vi "Serial RW.vi"(2 "Porta Serial":refnum<visa-resource-name>="COM7", 3 "Escrita":string, 4 "Função":u8) -> (0 "TemDado":bool, 1 "Leitura":string)   [LabVIEW 2012]
doc: "The Basic Serial Read and Write example performs a Serial Port Read, a Serial Port Write, or a combination of these actions. The user selects the actions (read or write) on the front panel. If both are selected, the VI will write the data first, read data, and then close the VISA session that is opened to the port. This VI will wait until the specified number of bytes is received at the port. Only the number of bytes specified will be read.\n\nINSTRUCTIONS:\n1) Select the serial resource and configuration parameters (baud rate, data bits, parity, stop bits, flow control).\n2) Select the operations to be performed. \n3) Connect the serial port to your device. If no device is available, perform a loopback test by doing one of the following. Short pins 2 and 3 on a RS-232 cable or short pin 4 to pin 8 and pin 5 to pin 9 on a RS-485/422 cable. \n4) Run the VI to see the data read. (The \"read string\" will match the \"string to write\" if a loopback test was performed.)\n\nNote: The parameters set for the serial port must match the parameters of the connected instrument or device. In this example, the bytes to read parameter specifies the number of bytes that the serial port reads. If there were more bytes at the port than the number specified in bytes to read, those bytes would not be read. Also, if you specify to read more bytes than the number of bytes actually read, you might receive a timeout error message.\n\nOn the block diagram, the Configure Serial Port VI sets the configuration parameters. The front panel displays the controls used to configure the basic parameters, such as baud rate, data bits, and parity. Constants configure the other parameters the user probably does not need set. After the VISA Configure Serial Port VI opens the VISA session and configures the port, the VI passes the VISA resource name to other VIs that perform operations on that VISA resource. The VISA Write function sends a command to the serial device and the VISA Read function returns data based on the command. The VISA Close function then closes the reference to the serial device. It is important to close the reference; otherwise communication through with that port through protocols other than VISA might not be possible."
uses:
  <vilib>/Instr/_visa.llb/VISA Configure Serial Port (Instr).vi
panel:
  out "bytes read":u32
  in  "error in":errorcluster
  in  "flow control":u16(ring) items=["None"=0, "XON/XOFF"=1, "RTS/CTS"=2, "DTR/DSR"=4]
  in  "stop bits":u16(ring)=10 items=["1.0"=10, "1.5"=15, "2.0"=20]
  in  "parity":u16(ring) items=["None", "Odd", "Even", "Mark", "Space"]
  in  "data bits":u16=8 min=5 max=8 step=1
  in  "baud rate":u32=9600
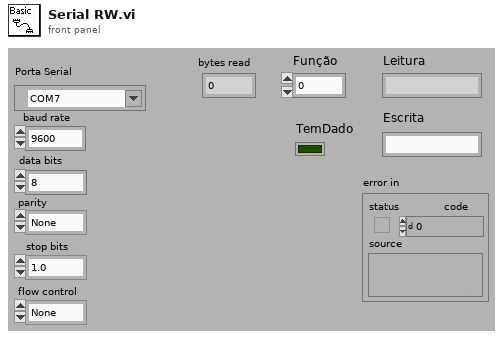
[diagram p1: front panel]
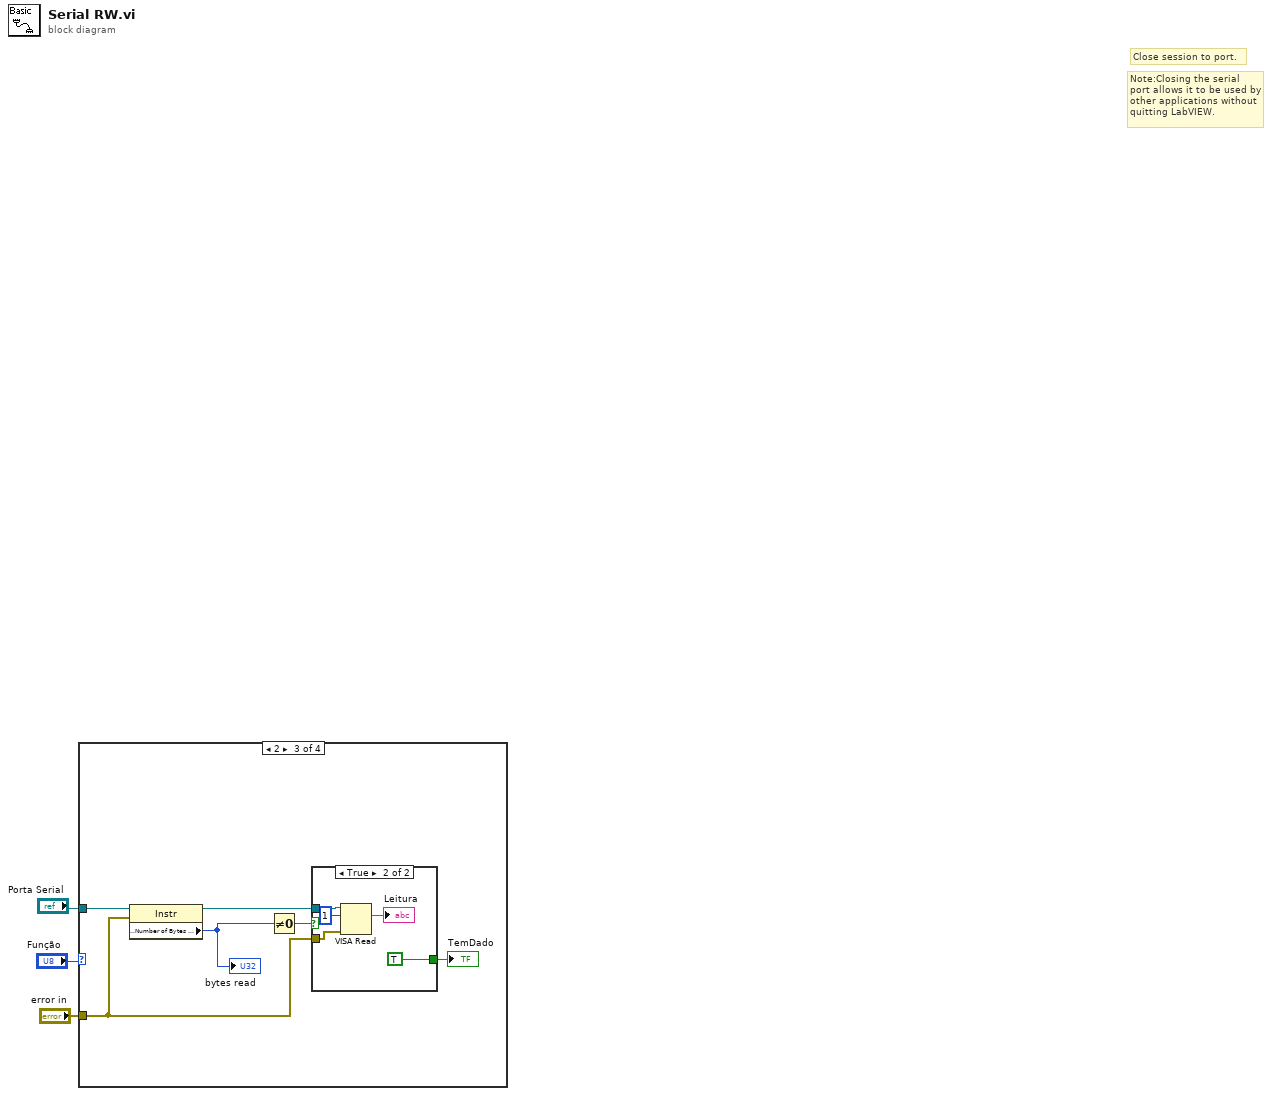
[diagram p0: block diagram]
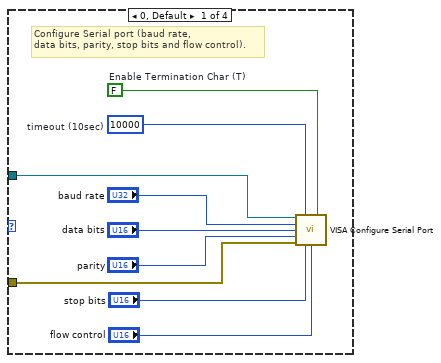
[diagram p2: hidden frame]
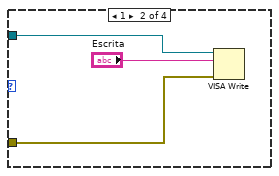
[diagram p3: hidden frame]
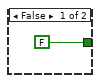
[diagram p4: hidden frame]
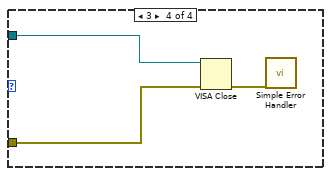
[diagram p5: hidden frame]
diagram:
  # "Note:Closing the serial port allows it to be used by other applications without\nquitting LabVIEW."
  # "Close session to port."
  n1 = case shown="2" "Função" {
    tunnel: "Porta Serial" -> [w5 w15 w21 w29]
    tunnel: "error in" -> [w4 w14 w16 w28]
    frame 0, Default {
      w9 = FALSE  # Enable Termination Char (T)
      w10 = u32 10000  # timeout (10sec)
      # "Configure Serial port (baud rate,\ndata bits, parity, stop bits and flow control)."
      n2 = call-poly "VISA Configure Serial Port"("VISA resource name"=w5, "timeout (10sec)"=w10, "Enable Termination\nChar (T)"=w9, "baud rate (9600)"="baud rate", "data bits (8)"="data bits", "parity (0:none)"="parity", "error in (no error)"=w4, "stop bits (10: 1 bit)"="stop bits", "flow control (0:none)"="flow control") -> ()  [unwired: 5 in, 2 out]
    }
    frame 1 {
      n3 = VISA Write(VISA resource name=w15, write buffer="Escrita", error in (no error)=w14) -> ()  [unwired: 3 out]
    }
    frame 2 {
      n4 = property class="Instr"(reference=w21, error in=w16) -> (reference out=w18:refnum<visa-resource-name>, "Serial Settings:Number of Bytes at Serial Port"=w19:u32)  [unwired: 1 out]
      "bytes read" <- w19
      n5 = Not Equal To 0?(x=w19) -> (x != 0?=w20:bool)
      n6 = case shown="True" w20 {
        tunnel: w18 -> [_ w27]
        tunnel: w16 -> [_ w26]
        tunnel: [FALSE ("TemDado") TRUE ("TemDado")] -> w17
        frame False {
        }
        frame True {
          n7 = VISA Read(VISA resource name=w27, byte count=u32 1, error in (no error)=w26) -> (read buffer=→"Leitura":string)  [unwired: 3 out]
        }
      }
      "TemDado" <- w17
    }
    frame 3 {
      n8 = VISA Close(VISA resource name=w29, error in (no error)=w28) -> (error out=w30:errorcluster)
      n9 = call <vilib>:"Simple Error Handler.vi"("error in (no error)"=w30) -> ()  [unwired: 4 in, 5 out]
    }
  }
